vi "readFromXML.vi"(8 "error in (no error)":errorcluster, 10 "XML in":string, 11 "OffsetStatus in":refnum<class "OffsetStatus.lvclass">) -> (0 "error out":errorcluster, 3 "OffsetStatus out":refnum<class "OffsetStatus.lvclass">)   [LabVIEW 2014, in "TCSDataDefinitions.lvlib" / "TCSPublicStatus.lvlib" / "OffsetStatus.lvclass"]
uses:
  OffsetStatus.lvclass
  TCSCommand/OffsetCommands/OffsetDef/Enumerations/OffsetType.ctl
  <userlib>/Common/UnitsAndXML/FlattenItemWithUnitToXML/FlattenTimeToXML/TimeUnit.ctl
  <userlib>/Common/UnitsAndXML/FlattenItemWithUnitToXML/FlattenPlaneAngleToXML/PlaneAngleUnit.ctl
  OffsetStatus.lvclass/OffsetStatus.ctl
  <userlib>/Common/UnitsAndXML/UnitsAndXML.lvlib
  <userlib>/Common/XML/XMLParser/XMLParser.lvclass
  TCSCommand/OffsetCommands/OffsetCommands.lvlib
panel:
  out "handsetOff2":dbl[unit]
  out "handsetOff1":dbl[unit]
  out "userOff2":dbl[unit]
  out "userOff1":dbl[unit]
  out "offsetType":T1
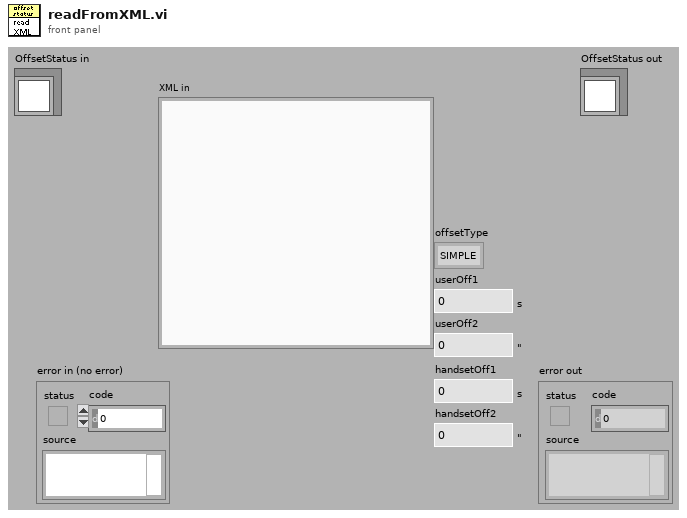
[diagram p1: front panel]
types:
  T1 = typedef "TCSDataDefinitions.lvlib/TCSCommand.lvlib/OffsetCommands.lvlib/OffsetType.ctl" = enum16{"SIMPLE", "TPLANE", "PA"}
  T2 = typedef "UnitsAndXML.lvlib/PlaneAngleUnit.ctl" = enum16{"rad", "deg", "'", "\""}
  T3 = typedef "UnitsAndXML.lvlib/TimeUnit.ctl" = enum16{"s", "d", "h", "min", "a"}
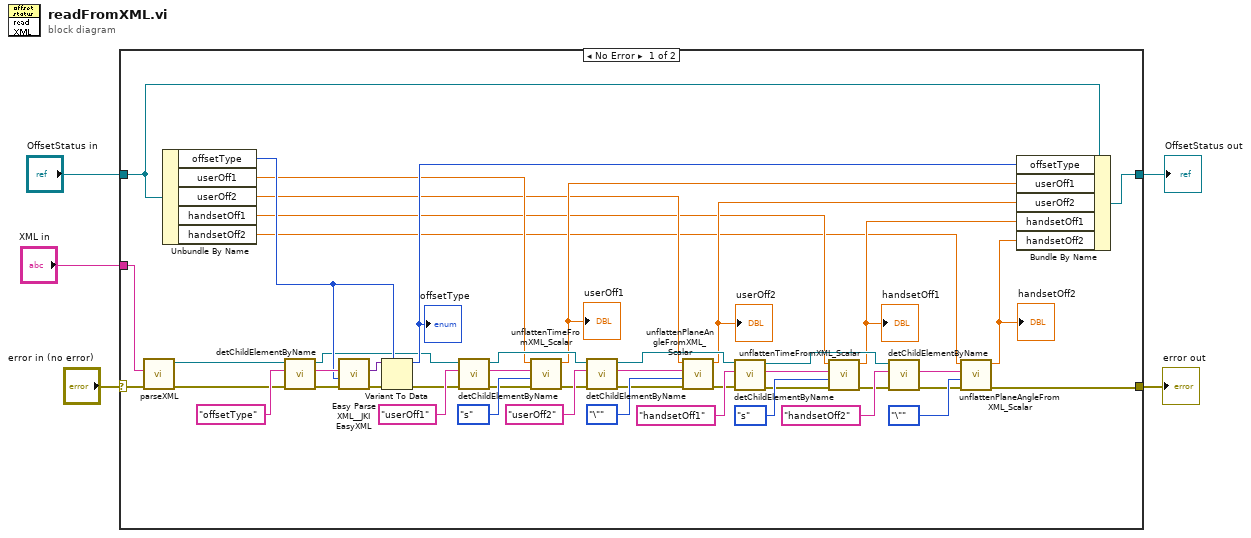
[diagram p0: block diagram]
diagram:
  n1 = case shown="No Error" "error in (no error)" {
    selector: "error in (no error)" -> [w50 w53]
    tunnel: [w49 w52] -> w2
    tunnel: "OffsetStatus in" -> [w41 w52]
    tunnel: "XML in" -> [w51 _]
    tunnel: [w18 w53] -> w3
    frame No Error {
      n2 = call <userlib>:"parseXML.vi"("error in (no error)"=w50, "XMLString in"=w51) -> ("error out"=w6:errorcluster, "Element out"=w7:refnum<class "XMLParser.lvclass">)  [unwired: 8 in]
      n3 = Unbundle By Name(w41) -> ("offsetType"=w44:T1, "userOff1"=w11:dbl[unit], "userOff2"=w10:dbl[unit], "handsetOff1"=w9:dbl[unit], "handsetOff2"=w8:dbl[unit])
      n4 = call <userlib>:"detChildElementByName.vi"("error in (no error)"=w6, "childName"="offsetType" ("ChildName"), "Element in"=w7) -> ("error out"=w42:errorcluster, "childXML"=w45:string, "Element out"=w17:refnum<class "XMLParser.lvclass">)  [unwired: 5 in, 1 out]
      n5 = call <vilib>:"Easy Parse XML__JKI EasyXML.vi"("error in (no error)"=w42, "LabVIEW Data (Type)"=w44, "XML String"=w45) -> ("error out"=w47:errorcluster, "LabVIEW Data"=w46:variant)  [unwired: 7 in]
      n6 = Variant To Data(error in=w47, type=w44, Variant=w46) -> (data=w43:T1, error out=w20:errorcluster)
      "offsetType" <- w43
      n7 = call <userlib>:"detChildElementByName.vi"("error in (no error)"=w20, "childName"="userOff1" ("ChildName"), "Element in"=w17) -> ("error out"=w36:errorcluster, "childXML"=w38:string, "Element out"=w31:refnum<class "XMLParser.lvclass">)  [unwired: 5 in, 1 out]
      n8 = call <userlib>:"unflattenTimeFromXML_Scalar.vi"("error in (no error)"=w36, "timeUnitInXML"=TimeUnit."s", "xmlString"=w38, "timeForType"=w11) -> ("error out"=w35:errorcluster, "time"=w15:dbl[unit])  [unwired: 6 in]
      "userOff1" <- w15
      n9 = call <userlib>:"detChildElementByName.vi"("error in (no error)"=w35, "childName"="userOff2" ("ChildName"), "Element in"=w31) -> ("error out"=w32:errorcluster, "childXML"=w34:string, "Element out"=w16:refnum<class "XMLParser.lvclass">)  [unwired: 5 in, 1 out]
      n10 = call <userlib>:"unflattenPlaneAngleFromXML_Scalar.vi"("error in (no error)"=w32, "planeAngleUnitInXML"=PlaneAngleUnit."\"", "xmlString"=w34, "planeAngleForType"=w10) -> ("error out"=w19:errorcluster, "planeAngle"=w14:dbl[unit])  [unwired: 6 in]
      "userOff2" <- w14
      n11 = call <userlib>:"detChildElementByName.vi"("error in (no error)"=w19, "childName"="handsetOff1" ("ChildName"), "Element in"=w16) -> ("error out"=w26:errorcluster, "childXML"=w28:string, "Element out"=w21:refnum<class "XMLParser.lvclass">)  [unwired: 5 in, 1 out]
      n12 = call <userlib>:"unflattenTimeFromXML_Scalar.vi"("error in (no error)"=w26, "timeUnitInXML"=TimeUnit."s", "xmlString"=w28, "timeForType"=w9) -> ("error out"=w25:errorcluster, "time"=w13:dbl[unit])  [unwired: 6 in]
      "handsetOff1" <- w13
      n13 = call <userlib>:"detChildElementByName.vi"("error in (no error)"=w25, "childName"="handsetOff2" ("ChildName"), "Element in"=w21) -> ("error out"=w22:errorcluster, "childXML"=w24:string)  [unwired: 5 in, 2 out]
      n14 = call <userlib>:"unflattenPlaneAngleFromXML_Scalar.vi"("error in (no error)"=w22, "planeAngleUnitInXML"=PlaneAngleUnit."\"", "xmlString"=w24, "planeAngleForType"=w8) -> ("error out"=w18:errorcluster, "planeAngle"=w12:dbl[unit])  [unwired: 6 in]
      "handsetOff2" <- w12
      n15 = Bundle By Name(cluster=w41, "offsetType"=w43, "userOff1"=w15, "userOff2"=w14, "handsetOff1"=w13, "handsetOff2"=w12) -> (w49:refnum<class "OffsetStatus.lvclass">)
    }
    frame Error {
    }
  }
  "error out" <- w3
  "OffsetStatus out" <- w2
